vi "set_v.vi"(8 "error in (no error)":errorcluster, 9 "Voltage (V)":dbl, 10 "Channel":string="1", 11 "VISA Refnum in":refnum<visa-resource-name>) -> (0 "error out":errorcluster, 3 "VISA Refnum out":refnum<visa-resource-name>)   [LabVIEW 2018, in "Aim-TTi PL303-P.lvlib"]
uses:
  <instrlib>/Aim-TTi PL303-P/Aim-TTi PL303-P.lvlib
panel:
  out "concatenated string":string
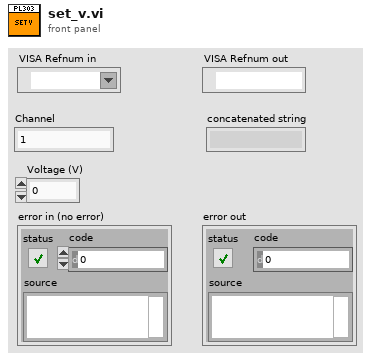
[diagram p1: front panel]
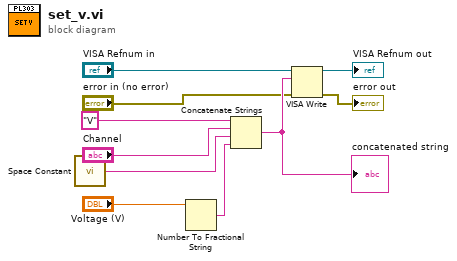
[diagram p0: block diagram]
diagram:
  n1 = call <vilib>:"Space Constant.vi"() -> ("String"=w3:string)
  n2 = Number To Fractional String(number="Voltage (V)") -> (F-format string=w1:string)  [unwired: 3 in]
  n3 = Concatenate Strings("V" ("string"), "Channel", w3, w1) -> (w8:string)
  "concatenated string" <- w8
  n4 = VISA Write(VISA resource name="VISA Refnum in", write buffer=w8, error in (no error)="error in (no error)") -> (VISA resource name out=→"VISA Refnum out":refnum<visa-resource-name>, error out=→"error out":errorcluster)  [unwired: 1 out]
